vi "GetDocumentTitle.vi"(0 "reference in":refnum<class "DP_WebView.lvclass">, 5 "Error In":errorcluster) -> (14 "reference out":refnum<class "DP_WebView.lvclass">, 15 "DocumentTitle":string, 19 "Error Out":errorcluster)   [LabVIEW 2020, in "DP_WebView.lvclass"]
doc: "Get Document Ttile"
uses:
  DP_WebView.lvclass
  C:/Projects/DependencyViewer/DependencyViewer/DP_WebView_class/data/Microsoft.Web.WebView2.Core.dll
  data/Microsoft.Web.WebView2.Core.dll
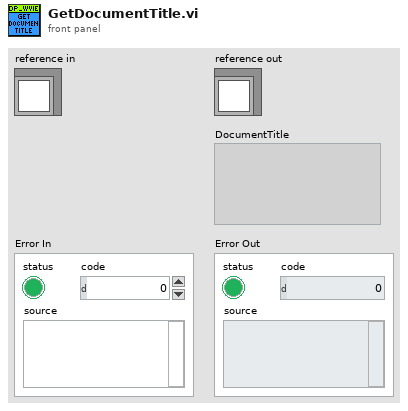
[diagram p1: front panel]
types:
  T1 = typedef "DP_WebView.lvclass/ObjectAttributes.ctl" = cluster{"WebView Container":refnum<k24>, "CoreWebViewRef":refnum<k24>, "Status":i32, "Status Message":string, "User Data Folder":path, "BrowserProcessId":u32}
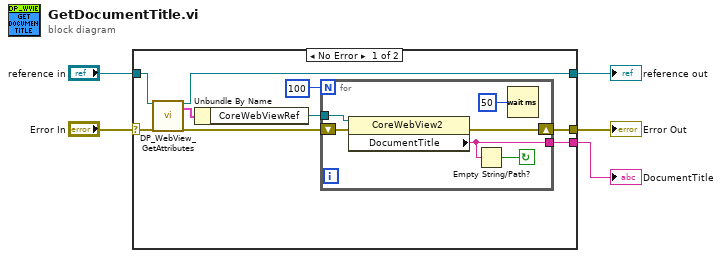
[diagram p0: block diagram]
diagram:
  n1 = case shown="No Error" "Error In" {
    selector: "Error In" -> [w14 w22]
    tunnel: [w8 w22] -> w4
    tunnel: [w11 w21] -> w2
    tunnel: "reference in" -> [w12 w21]
    tunnel: [w7 _] -> w1
    frame No Error {
      n2 = call "DP_WebView_GetAttributes.vi"("reference in"=w12, "error in (no error)"=w14) -> ("reference out"=w11:refnum<class "DP_WebView.lvclass">, "Data"=w13:T1, "error out"=w9:errorcluster)  [unwired: 14 in, 1 out]
      n3 = Unbundle By Name(w13) -> ("CoreWebViewRef"=w10:refnum<k24>)
      n4 = for {
        N: 100 -> [_]
        tunnel: w10 -> [w20]
        tunnel: [w17] -> w7
        shift-right: [w18] -> w8
        shift-left: w9 -> [w19]
        stop <- w16 continue-if-true
        n5 = property class="CoreWebView2"(reference=w20, error in=w19) -> (error out=w18:errorcluster, "DocumentTitle"=w17:string)  [unwired: 1 out]
        n6 = Empty String/Path?(string/path=w17) -> (empty?=w16:bool)
        n7 = Wait (ms)(milliseconds to wait=u32 50) -> ()  [unwired: 1 out]
      }
    }
    frame Error {
    }
  }
  "Error Out" <- w4
  "reference out" <- w2
  "DocumentTitle" <- w1
